vi "室外图片保存.vi"(10 "路径":path) -> ()   [LabVIEW 2018]
panel:
  out "视频帧数":u32
  in  "数据输入界限:最大值":dbl
  in  "下一步":bool
  in  "?":bool
  out "?":T1(plugin-control)
  in  "选择需要保存的帧数":u32=1 min=1 max=241
  in  "停止":bool
  # "图片保存"
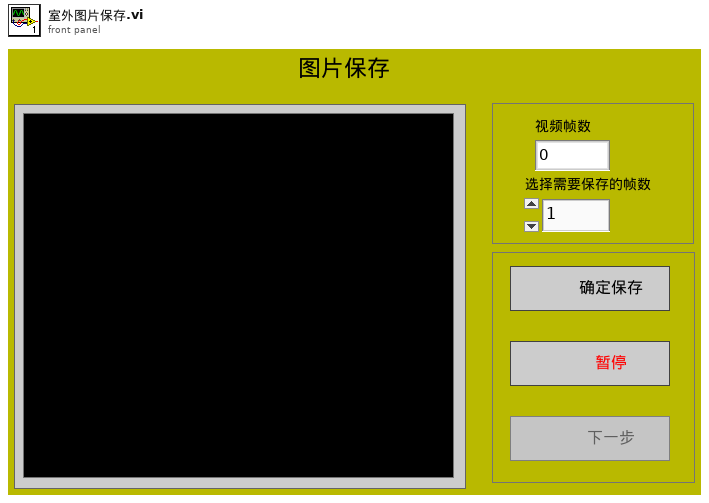
[diagram p1: front panel]
types:
  T1 = typedef "IMAQ Image.ctl" = refnum<image>
  T2 = typedef "Image Type" = u32
  T3 = enum32{"Invalid", "Standard", "Closed", "Hidden", "Minimized", "Maximized"}
  T4 = enum8{"Enabled", "Disabled", "Disabled and Grayed Out"}
  T5 = typedef "IMAQ AVI2 Refnum.ctl" = refnum<k20>
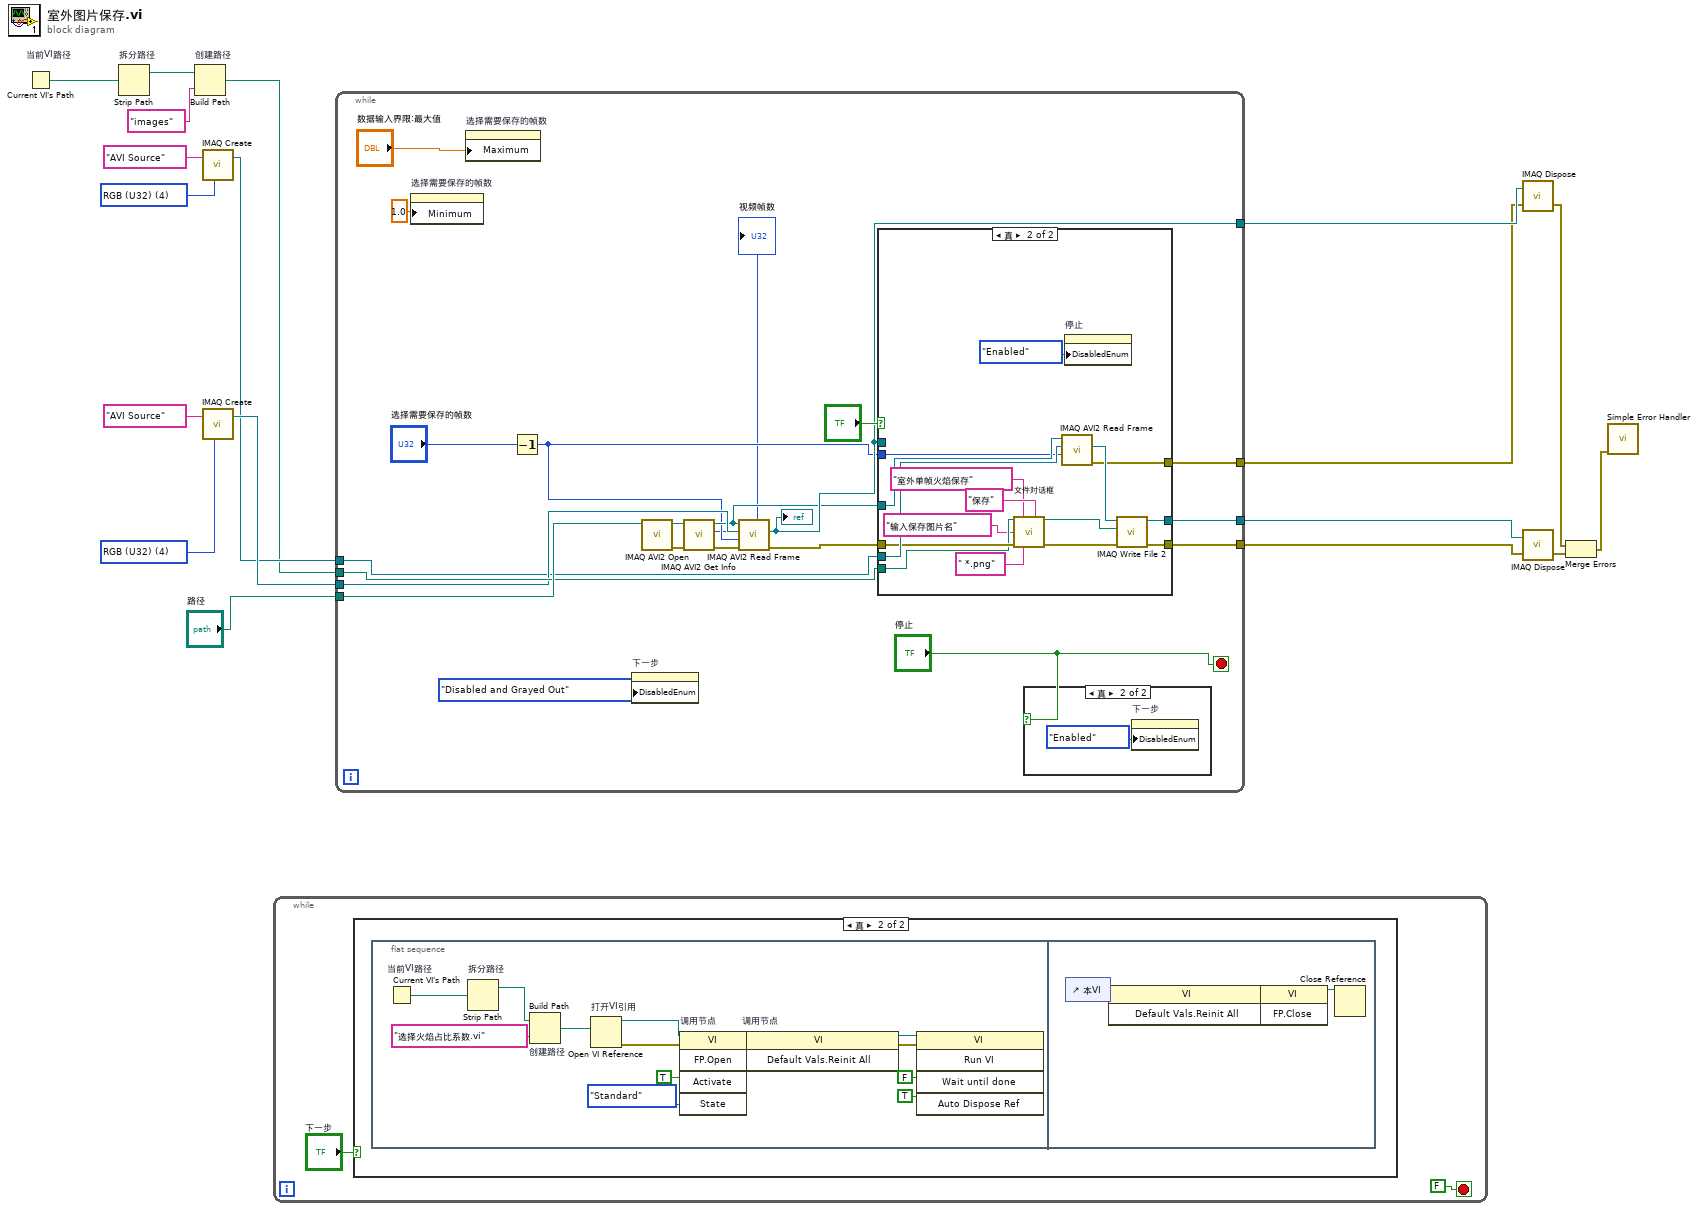
[diagram p0: block diagram]
diagram:
  w12 = T2 4 items=["Grayscale (U8)", "Grayscale (I16)", "Grayscale (SGL)", "Complex (CSG)", "RGB (U32)", "HSL (U32)", "RGB (U64)", "Grayscale (U16)"] ("Image Type")
  w5 = T2 4 items=["Grayscale (U8)", "Grayscale (I16)", "Grayscale (SGL)", "Complex (CSG)", "RGB (U32)", "HSL (U32)", "RGB (U64)", "Grayscale (U16)"] ("Image Type")
  n1 = Current VI's Path "当前VI路径"() -> (path=w3:path)
  n2 = Strip Path "拆分路径"(path=w3) -> (stripped path=w4:path)  [unwired: 1 out]
  n3 = Build Path "创建路径"(base path=w4, name or relative path="images" ("名称或相对路径")) -> (appended path=w1:path)
  n4 = call "IMAQ Create"("Image Name"="AVI Source", "Image Type"=w12) -> ("New Image"=w13:T1)  [unwired: 2 in, 2 out]
  n5 = call "IMAQ Create"("Image Name"="AVI Source", "Image Type"=w5) -> ("New Image"=w16:T1)  [unwired: 2 in, 2 out]
  n6 = while {
    stop <- FALSE stop-if-true
    n7 = case shown="真" "下一步" {
      frame False {
      }
      frame True {
        n8 = flat-sequence {
          frame #0 {
            n9 = Current VI's Path "当前VI路径"() -> (path=w30:path)
            n10 = Strip Path "拆分路径"(path=w30) -> (stripped path=w34:path)  [unwired: 1 out]
            n11 = Build Path "创建路径"(base path=w34, name or relative path="选择火焰占比系数.vi" ("名称或相对路径")) -> (appended path=w31:path)
            n12 = Open VI Reference "打开VI引用"(vi path=w31) -> (vi reference=w29:refnum<vi>, error out=w28:errorcluster)  [unwired: 5 in]
            n13 = invoke on="调用节点" class="VI" method="FP.Open"(reference=w29, error in=w28, "Activate"=TRUE ("激活？"), "State"=T3."Standard" ("状态")) -> (reference out=w27:refnum<vi>, error out=w26:errorcluster)  [unwired: 1 in, 3 out]
            n14 = invoke on="调用节点" class="VI" method="Default Vals.Reinit All"(reference=w27, error in=w26) -> (reference out=w23:refnum<vi>, error out=w24:errorcluster)  [unwired: 1 in, 1 out]
            n15 = invoke class="VI" method="Run VI"(reference=w23, error in=w24, "Wait until done"=FALSE ("结束前等待"), "Auto Dispose Ref"=TRUE ("自动销毁引用")) -> ()  [unwired: 1 in, 5 out]
          }
          frame #1 {
            n16 = control-ref of="本VI"() -> (w37:refnum<vi>)
            n17 = invoke class="VI" method="Default Vals.Reinit All"(reference=w37) -> (reference out=w36:refnum<vi>)  [unwired: 2 in, 2 out]
            n18 = invoke class="VI" method="FP.Close"(reference=w36) -> (reference out=w35:refnum<vi>)  [unwired: 2 in, 2 out]
            n19 = Close Reference(reference=w35) -> ()  [unwired: 1 in, 1 out]
          }
        }
      }
    }
  }
  n20 = while {
    tunnel: "路径" -> [w57]
    tunnel: [w56] -> w11
    tunnel: [w54] -> w10
    tunnel: w1 -> [w53]
    tunnel: w16 -> [w52]
    tunnel: [w51] -> w15
    tunnel: w13 -> [w50]
    tunnel: [w47] -> w8
    stop <- "停止" stop-if-true
    n21 = property on="选择需要保存的帧数" class="DigNum (严格)"("Minimum"=1.0 ("数据输入界限:最小值")) -> ()  [unwired: 2 in, 2 out]
    n22 = property on="选择需要保存的帧数" class="DigNum (严格)"("Maximum"="数据输入界限:最大值") -> ()  [unwired: 2 in, 2 out]
    n23 = Decrement(x="选择需要保存的帧数") -> (x-1=w46:u32)
    n24 = property on="下一步" class="Bool"("DisabledEnum"=T4."Disabled and Grayed Out" ("禁用")) -> ()  [unwired: 2 in, 2 out]
    n25 = call "IMAQ AVI2 Open"("AVI File Path"=w57) -> ("error out"=w44:errorcluster, "AVI Refnum"=w43:T5)  [unwired: 2 in, 7 out]
    n26 = call "IMAQ AVI2 Get Info"("error in (no error)"=w44, "AVI Refnum"=w43) -> ("error out"=w42:errorcluster, "Number of Frames"=→"视频帧数":u32, "AVI Refnum (duplicate)"=w49:T5)  [unwired: 7 out]
    n27 = call "IMAQ AVI2 Read Frame"("error in (no error)"=w42, "Frame Number"=w46, "Image"=w52, "AVI Refnum"=w49) -> ("error out"=w55:errorcluster, "Image Out"=w51:T1)  [unwired: 6 out]
    "?" <- w51
    n28 = case shown="真" "?" {
      tunnel: w51 -> [_ _]
      tunnel: [_ w75] -> w56
      tunnel: w55 -> [_ w67]
      tunnel: [_ w74] -> w54
      tunnel: w53 -> [_ w65]
      tunnel: w50 -> [_ w73]
      tunnel: w49 -> [_ w72]
      tunnel: w46 -> [_ w71]
      tunnel: [_ w69] -> w47
      frame False {
      }
      frame True {
        n29 = call "文件对话框"("start path"=w65, "prompt"="室外单帧火焰保存", "button label"="保存", "default name"="输入保存图片名" ("prompt"), "error in"=w67, "pattern (all files)"=" *.png") -> ("selected path"=w68:path, "error out"=w66:errorcluster)  [unwired: 6 in, 2 out]
        n30 = call "IMAQ AVI2 Read Frame"("Frame Number"=w71, "Image"=w73, "AVI Refnum"=w72) -> ("error out"=w69:errorcluster, "Image Out"=w70:T1)  [unwired: 1 in, 6 out]
        n31 = property on="停止" class="Bool"("DisabledEnum"=T4."Enabled" ("禁用")) -> ()  [unwired: 2 in, 2 out]
        n32 = call-poly "IMAQ Write File 2"("error in (no error)"=w66, "File Path"=w68, "Image"=w70) -> ("error out"=w74:errorcluster, "Image Out (duplicate)"=w75:T1)  [unwired: 7 in]
      }
    }
    n33 = case shown="真" "停止" {
      frame False {
      }
      frame True {
        n34 = property on="下一步" class="Bool"("DisabledEnum"=T4."Enabled" ("禁用")) -> ()  [unwired: 2 in, 2 out]
      }
    }
  }
  n35 = call "IMAQ Dispose"("Image"=w15, "error in (no error)"=w8) -> ("error out"=w7:errorcluster)  [unwired: 4 in]
  n36 = call "IMAQ Dispose"("Image"=w11, "error in (no error)"=w10) -> ("error out"=w9:errorcluster)  [unwired: 4 in]
  n37 = Merge Errors(w7, w9) -> (w6:errorcluster)
  n38 = call <vilib>:"Simple Error Handler.vi"("error in (no error)"=w6) -> ()  [unwired: 4 in, 5 out]
